vi "Download and Unzip.vi"(8 "error in":errorcluster, 11 "download from path":path=path "\\\\Nirvana\\AE-General/Cullen Clark") -> (0 "error out":errorcluster, 1 "failed?":bool, 3 "downloaded path":path)   [LabVIEW 2018]
uses:
  <vilib>/Utility/sysdir.llb/System Directory Type.ctl
  <vilib>/zip/NI_Unzip.lvlib
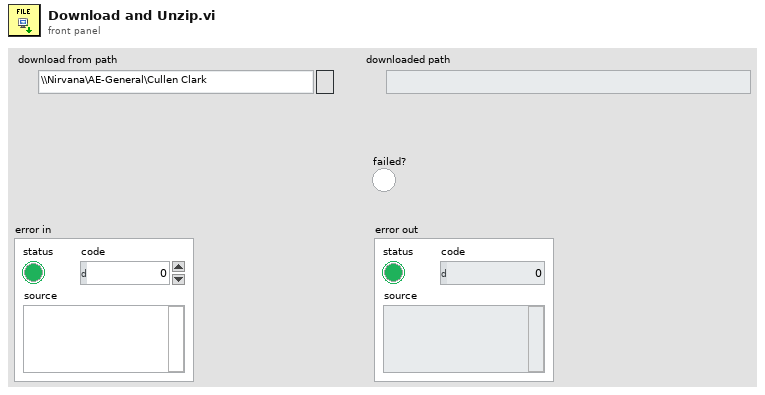
[diagram p1: front panel]
types:
  T1 = typedef "System Directory Type.ctl" = i32
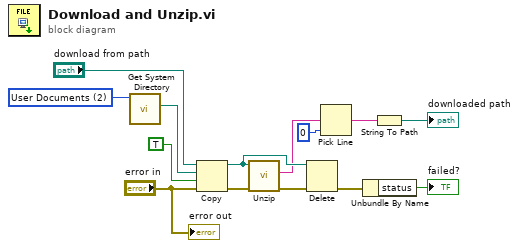
[diagram p0: block diagram]
diagram:
  w3 = T1 2 items=["User Home"=0, "User Desktop"=1, "User Documents"=2, "User Application Data"=3, "User Preferences"=4, "User Temporary"=5, "Public Documents"=6, "Public Application Data"=7, "Public Preferences"=8, "Public Cache"=13, "System Core Libraries"=9, "System Installed Libraries"=10, "Application Files"=11, "Boot Volume Root"=12] ("system directory type")
  n1 = call <vilib>:"Get System Directory.vi"("system directory type"=w3) -> ("system directory"=w2:path)  [unwired: 10 in]
  n2 = Copy(8:"error in", 9:TRUE ("overwrite (F)"), 10:w2, 11:"download from path") -> (0:w14:errorcluster, 3:w11:path)  [unwired: 1 in, 1 out]
  n3 = call <vilib>:"Unzip.vi"("error in (no error)"=w14, "Zip file"=w11) -> ("error out"=w12:errorcluster, "Preview"=w10:string)  [unwired: 7 in, 1 out]
  n4 = Delete(path (use dialog)=w11, error in=w12) -> (error out=w6:errorcluster)  [unwired: 3 in, 2 out]
  n5 = Pick Line(multi-line string=w10, line index=0) -> (output string=w8:string)  [unwired: 1 in]
  n6 = Unbundle By Name(w6) -> ("status"=→"failed?":bool)
  n7 = String To Path(string=w8) -> (path=→"downloaded path":path)
  "error out" <- "error in"
